vi "BinanceAPI_VI_TREE.vi"   [LabVIEW 2022 SP3, in "BinanceAPI_.lvclass"]
doc: "You should always us \"Start\" and \"Stop\" vi's, which initialize and close http connection. \nLook into Example.\n\nAbout methods look into Binance API documentation:\n - https://binance-docs.github.io/apidocs/\n\nAuthor tried imitate usualy used API function.\n\nWhite function is Spot used basic functions of Binance API.\nPurple function is Future used function with e.g. leverage options when you propably always will loose."
uses:
  BinanceAPI_.lvclass
panel:
  # "API  BINANCE \n    VI  TREE"
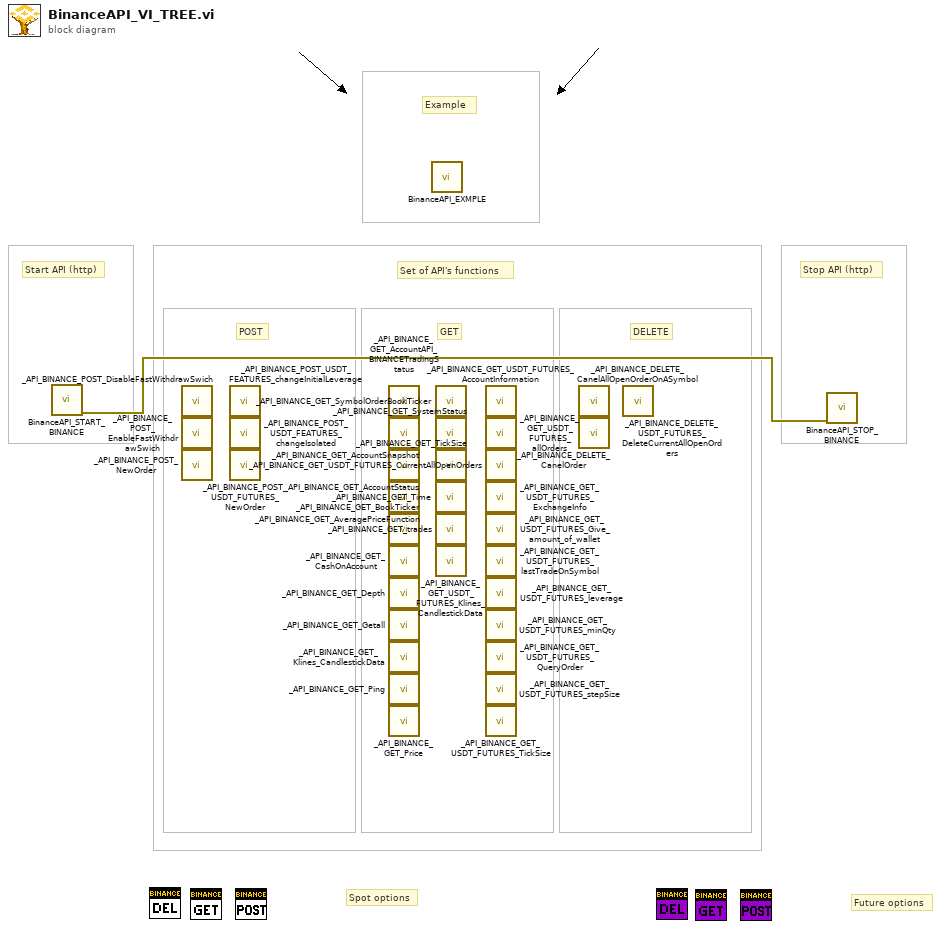
[diagram p0: block diagram]
diagram:
  # "Example"
  # "Spot options"
  # "Future options"
  # "DELETE"
  # "GET"
  # "POST"
  # "Set of API's functions"
  # "Stop API (http)"
  # "Start API (http)"
  n1 = call "BinanceAPI_START_BINANCE.vi"() -> ("error out"=w1:errorcluster)  [unwired: 13 in, 2 out]
  n2 = call "_API_BINANCE_POST_DisableFastWithdrawSwich.vi"() -> ()  [unwired: 13 in, 3 out]
  n3 = call "_API_BINANCE_POST_EnableFastWithdrawSwich.vi"() -> ()  [unwired: 13 in, 3 out]
  n4 = call "_API_BINANCE_POST_NewOrder.vi"() -> ()  [unwired: 13 in, 3 out]
  n5 = call "_API_BINANCE_POST_USDT_FEATURES_changeInitialLeverage.vi"() -> ()  [unwired: 13 in, 3 out]
  n6 = call "_API_BINANCE_POST_USDT_FEATURES_changeIsolated.vi"() -> ()  [unwired: 13 in, 3 out]
  n7 = call "_API_BINANCE_POST_USDT_FUTURES_NewOrder.vi"() -> ()  [unwired: 13 in, 3 out]
  n8 = call "_API_BINANCE_GET_AccountAPI_BINANCETradingStatus.vi"() -> ()  [unwired: 12 in, 4 out]
  n9 = call "_API_BINANCE_GET_AccountSnapshot.vi"() -> ()  [unwired: 12 in, 4 out]
  n10 = call "_API_BINANCE_GET_AccountStatus.vi"() -> ()  [unwired: 12 in, 4 out]
  n11 = call "_API_BINANCE_GET_AveragePriceFunction.vi"() -> ()  [unwired: 12 in, 4 out]
  n12 = call "_API_BINANCE_GET_BookTicker.vi"() -> ()  [unwired: 12 in, 4 out]
  n13 = call "_API_BINANCE_GET_CashOnAccount.vi"() -> ()  [unwired: 12 in, 4 out]
  n14 = call "_API_BINANCE_GET_Depth.vi"() -> ()  [unwired: 12 in, 4 out]
  n15 = call "_API_BINANCE_GET_Getall.vi"() -> ()  [unwired: 12 in, 4 out]
  n16 = call "_API_BINANCE_GET_Klines_CandlestickData.vi"() -> ()  [unwired: 12 in, 4 out]
  n17 = call "_API_BINANCE_GET_Ping.vi"() -> ()  [unwired: 12 in, 4 out]
  n18 = call "_API_BINANCE_GET_Price.vi"() -> ()  [unwired: 12 in, 4 out]
  n19 = call "BinanceAPI_EXMPLE.vi"() -> ()  [unwired: 1 in]
  n20 = call "_API_BINANCE_GET_SymbolOrderBookTicker.vi"() -> ()  [unwired: 12 in, 4 out]
  n21 = call "_API_BINANCE_GET_SystemStatus.vi"() -> ()  [unwired: 12 in, 4 out]
  n22 = call "_API_BINANCE_GET_TickSize.vi"() -> ()  [unwired: 13 in, 3 out]
  n23 = call "_API_BINANCE_GET_Time.vi"() -> ()  [unwired: 12 in, 4 out]
  n24 = call "_API_BINANCE_GET_trades.vi"() -> ()  [unwired: 12 in, 4 out]
  n25 = call "_API_BINANCE_GET_USDT_FUTURES_Klines_CandlestickData.vi"() -> ()  [unwired: 12 in, 4 out]
  n26 = call "_API_BINANCE_GET_USDT_FUTURES_AccountInformation.vi"() -> ()  [unwired: 12 in, 4 out]
  n27 = call "_API_BINANCE_GET_USDT_FUTURES_allOrders.vi"() -> ()  [unwired: 12 in, 4 out]
  n28 = call "_API_BINANCE_GET_USDT_FUTURES_CurrentAllOpenOrders.vi"() -> ()  [unwired: 13 in, 3 out]
  n29 = call "_API_BINANCE_GET_USDT_FUTURES_ExchangeInfo.vi"() -> ()  [unwired: 11 in, 5 out]
  n30 = call "_API_BINANCE_GET_USDT_FUTURES_Give_amount_of_wallet.vi"() -> ()  [unwired: 10 in, 6 out]
  n31 = call "_API_BINANCE_GET_USDT_FUTURES_lastTradeOnSymbol.vi"() -> ()  [unwired: 12 in, 4 out]
  n32 = call "_API_BINANCE_GET_USDT_FUTURES_leverage.vi"() -> ()  [unwired: 12 in, 4 out]
  n33 = call "_API_BINANCE_GET_USDT_FUTURES_minQty.vi"() -> ()  [unwired: 13 in, 3 out]
  n34 = call "_API_BINANCE_GET_USDT_FUTURES_QueryOrder.vi"() -> ()  [unwired: 13 in, 3 out]
  n35 = call "_API_BINANCE_GET_USDT_FUTURES_stepSize.vi"() -> ()  [unwired: 13 in, 3 out]
  n36 = call "_API_BINANCE_GET_USDT_FUTURES_TickSize.vi"() -> ()  [unwired: 12 in, 4 out]
  n37 = call "_API_BINANCE_DELETE_CanelAllOpenOrderOnASymbol.vi"() -> ()  [unwired: 13 in, 3 out]
  n38 = call "_API_BINANCE_DELETE_CanelOrder.vi"() -> ()  [unwired: 13 in, 3 out]
  n39 = call "_API_BINANCE_DELETE_USDT_FUTURES_DeleteCurrentAllOpenOrders.vi"() -> ()  [unwired: 13 in, 3 out]
  n40 = call "BinanceAPI_STOP_BINANCE.vi"("error in (no error)"=w1) -> ()  [unwired: 14 in, 1 out]
